vi "Is This Control Of This LabVIEW Class.vi"(8 "error in (no error)":errorcluster, 10 "LVClass Refnum":refnum<vi>, 11 "Ctl Refnum":refnum<vi>) -> (0 "error out":errorcluster, 1 "Is this control of this class?":bool, 2 "LVClass Refnum out":refnum<vi>, 3 "Ctl Refnum out":refnum<vi>)   [LabVIEW 2017]
doc: "Given a control refnum and a LVClass refnum, this VI determines whether the control is a control of the LVClass type. The VI will return true for the LVClass' regular class controls/indicators and for XControls whose type is the given LVClass. \n\nThis VI will return a \"not supported\" error in built applications."
uses:
  <vilib>/Utility/VariantDataType/VariantType.lvlib
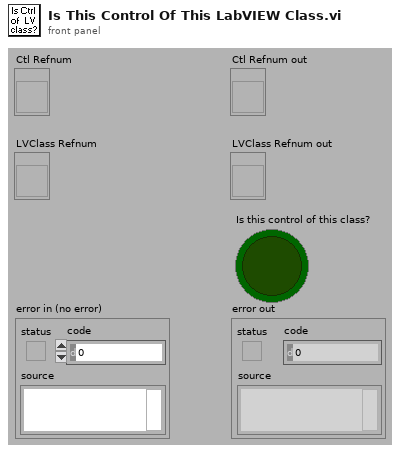
[diagram p1: front panel]
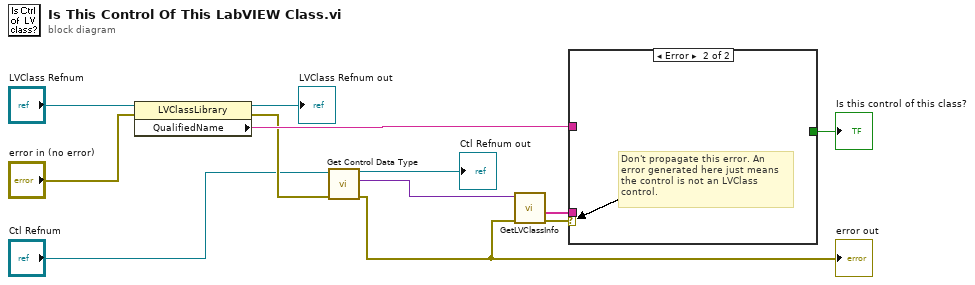
[diagram p0: block diagram]
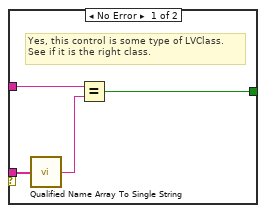
[diagram p2: hidden frame]
diagram:
  n1 = property class="LVClassLibrary"(reference="LVClass Refnum", error in="error in (no error)") -> (reference out=→"LVClass Refnum out":refnum<vi>, error out=w6:errorcluster, "QualifiedName"=w8:string)
  n2 = call <vilib>:"Get Control Data Type.vi"("error in (no error)"=w6, "Control Refnum in"="Ctl Refnum") -> ("error out"=w2:errorcluster, "Control's Data Type"=w11:variant, "Control Refnum out"=→"Ctl Refnum out":refnum<vi>)  [unwired: 3 in]
  "error out" <- w2
  n3 = call <vilib>:"GetLVClassInfo.vi"("error in (no error)"=w2, "Variant"=w11) -> ("error out"=w9:errorcluster, "Fully Qualified LV Class Name"=w10:string[])  [unwired: 7 in, 1 out]
  n4 = case shown="Error" w9 {
    tunnel: w10 -> [w16 _]
    tunnel: [w13 _] -> w12
    tunnel: w8 -> [w14 _]
    frame No Error {
      # "Yes, this control is some type of LVClass. \nSee if it is the right class."
      n5 = call <vilib>:"Qualified Name Array To Single String.vi"("Fully Qualified Array"=w16) -> ("Fully Qualified String"=w15:string)
      n6 = Equal?(x=w14, y=w15) -> (x = y?=w13:bool)
    }
    frame Error {
      # "Don't propagate this error. An error generated here just means the control is not an LVClass control."
    }
  }
  "Is this control of this class?" <- w12
